vi "Fetch Multi Eval Meas Trace ACLR Results.vi"(8 "error in (no error)":errorcluster, 9 "Result Type (Current)":i32(ring) items=["Current", "Average"], 10 "Instance (1)":T2=1, 11 "VISA resource name":refnum<visa-resource-name>) -> (0 "error out":errorcluster, 1 "ACLR Results":T1 {"NR Positive" format="%^.3e"; "NR Negative" format="%^.3e"; "UTRA 2 Positive" format="%^.3e"; "UTRA 1 Positive" format="%^.3e"; "Carrier" format="%^.3e"; "UTRA 1 Negative" format="%^.3e"; "UTRA 2 Negative" format="%^.3e"}, 2 "Reliability":i32, 3 "VISA resource name out":refnum<visa-resource-name>)   [LabVIEW 2020, in "Rohde&Schwarz CMWXP NR FR1 Measurement.lvlib"]
doc: "Returns the absolute powers as displayed in the ACLR diagram for NR standalone. The current and average values can be retrieved.\n\nAttributes:\nRSCMWXPNRFR1M_ATTR_FETCH_MULTI_EVAL_MEAS_TRACE_ACLR_CURRENT_RESULTS\nRSCMWXPNRFR1M_ATTR_FETCH_MULTI_EVAL_MEAS_TRACE_ACLR_AVERAGE_RESULTS\n\nRemote-control commands:\nFETCh:NRSub:MEAS<i>:MEValuation:TRACe:ACLR:CURRent?\nFETCh:NRSub:MEAS<i>:MEValuation:TRACe:ACLR:AVERage?"
uses:
  <instrlib>/Rohde&Schwarz CMWXP NR FR1 Measurement/Rohde&Schwarz CMWXP NR FR1 Measurement.lvlib
  <instrlib>/Rohde&Schwarz CMWXP NR FR1 Measurement/Private/_Instance.ctl
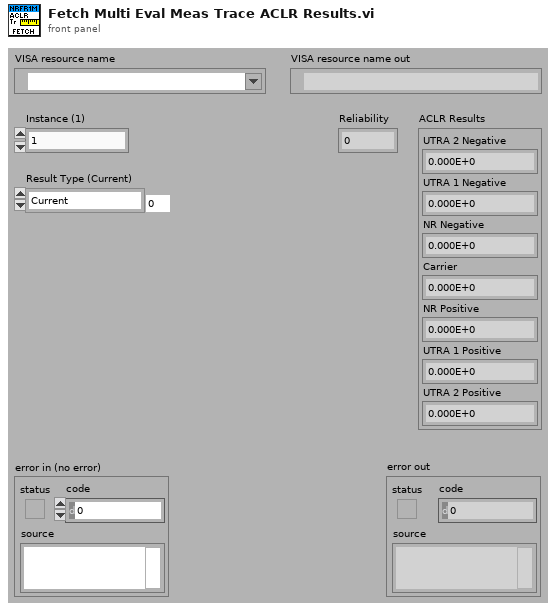
[diagram p1: front panel]
types:
  T1 = cluster{"UTRA 2 Negative":dbl, "UTRA 1 Negative":dbl, "NR Negative":dbl, "Carrier":dbl, "NR Positive":dbl, "UTRA 1 Positive":dbl, "UTRA 2 Positive":dbl}
  T2 = typedef "Rohde&Schwarz CMWXP NR FR1 Measurement.lvlib/_Instance.ctl" = i32
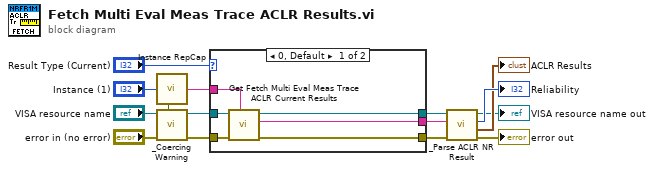
[diagram p0: block diagram]
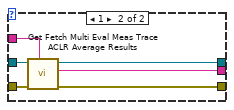
[diagram p2: hidden frame]
diagram:
  n1 = call <instrlib>:"Instance RepCap.vi"("Instance In"="Instance (1)") -> ("In Range?"=w13:bool, "RepCap Identifier Out"=w9:string)  [unwired: 1 in]
  n2 = call <instrlib>:"_Coercing Warning.vi"("In Range?"=w13, "error in (no error)"="error in (no error)", "VISA resource name"="VISA resource name") -> ("error out"=w10:errorcluster, "VISA resource name out"=w11:refnum<visa-resource-name>)  [unwired: 7 in]
  n3 = case shown="0, Default" "Result Type (Current)" {
    tunnel: w11 -> [w21 w27]
    tunnel: w10 -> [w20 w26]
    tunnel: w9 -> [w19 w25]
    tunnel: [w18 w24] -> w7
    tunnel: [w17 w23] -> w6
    tunnel: [w16 w22] -> w5
    frame 0, Default {
      n4 = call "Get Fetch Multi Eval Meas Trace ACLR Current Results"("Repeated Capabilities"=w19, "error in (no error)"=w20, "instrument handle"=w21) -> ("error out"=w18:errorcluster, "Fetch Multi Eval Meas Trace ACLR Current Results"=w16:string, "instrument handle out"=w17:refnum<visa-resource-name>)  [unwired: 6 in]
    }
    frame 1 {
      n5 = call "Get Fetch Multi Eval Meas Trace ACLR Average Results"("Repeated Capabilities"=w25, "error in (no error)"=w26, "instrument handle"=w27) -> ("error out"=w24:errorcluster, "Fetch Multi Eval Meas Trace ACLR Average Results"=w22:string, "instrument handle out"=w23:refnum<visa-resource-name>)  [unwired: 6 in]
    }
  }
  n6 = call <instrlib>:"_Parse ACLR NR Result.vi"("error in (no error)"=w7, "Input String"=w5, "VISA resource name"=w6) -> ("error out"=→"error out":errorcluster, "ACLR Results"=→"ACLR Results":T1, "Reliability"=→"Reliability":i32, "VISA resource name out"=→"VISA resource name out":refnum<visa-resource-name>)  [unwired: 5 in]
